vi "Change in Custom Actions.vi"(8 "error in (no error)":errorcluster, 10 "Custom Actions":T1[](array[typedef]), 11 "Bundle Builder in":refnum<class "Bundle Builder.lvclass">) -> (0 "error out":errorcluster, 1 "Custom Actions File Names":string[](array[string]), 2 "Product List File Names":string[](array[string]), 3 "Bundle Builder out":refnum<class "Bundle Builder.lvclass">, 4 "Bundle Filename":string)   [LabVIEW 2020, in "Bundle Builder.lvclass"]
uses:
  Bundle Builder.lvclass
  Typedef/Custom Action.ctl
  Bundle Builder.lvclass/Bundle Builder.ctl
  4f63f28f-5265-4602-8317-7e5f909f2807.vi
  5d65ce95-3f27-4ad9-b4d3-753b2ea8e44f.vi
  <vilib>/Comparison/Equal/Equal Functor/Equal Functor.lvclass
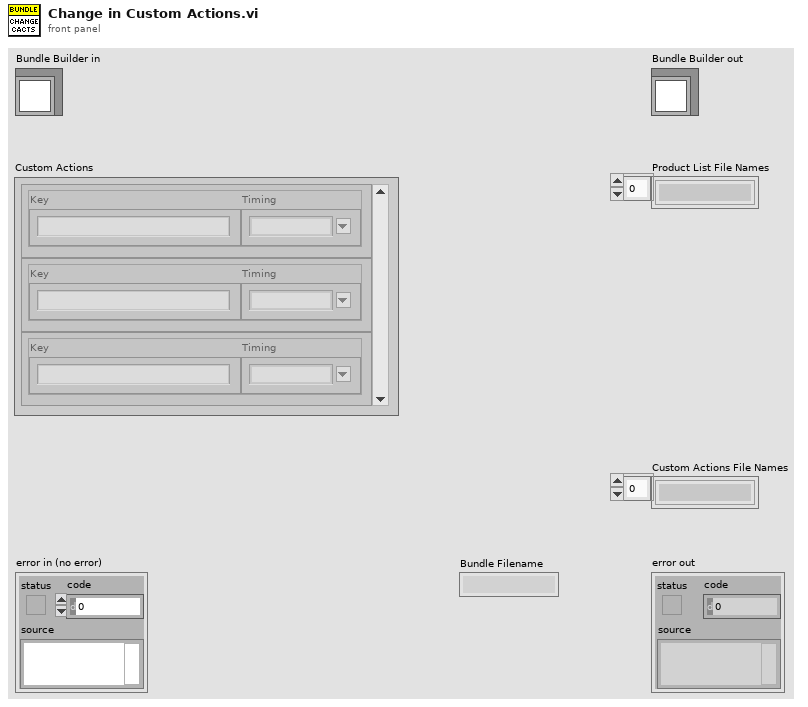
[diagram p1: front panel]
types:
  T1 = typedef "Custom Action.ctl" = cluster{"Key":string, "Timing":string}
  T2 = enum16{"All Elements Deleted", "Element Deleted", "Element Inserted", "Element Content Changed"}
  T3 = cluster{"Display Name":string, "Commands":cluster{"Path":string, "Parameters":string, "Successful Exit Codes":string}[]}[]
  T4 = cluster{"Display Name":string, "Commands":cluster{"Path":string, "Parameters":string, "Successful Exit Codes":string}[]}
  T5 = typedef "Custom Action Definition.ctl" = cluster{"Display Name":string, "Commands":cluster{"Path":string, "Parameters":string, "Successful Exit Codes":string}[]}
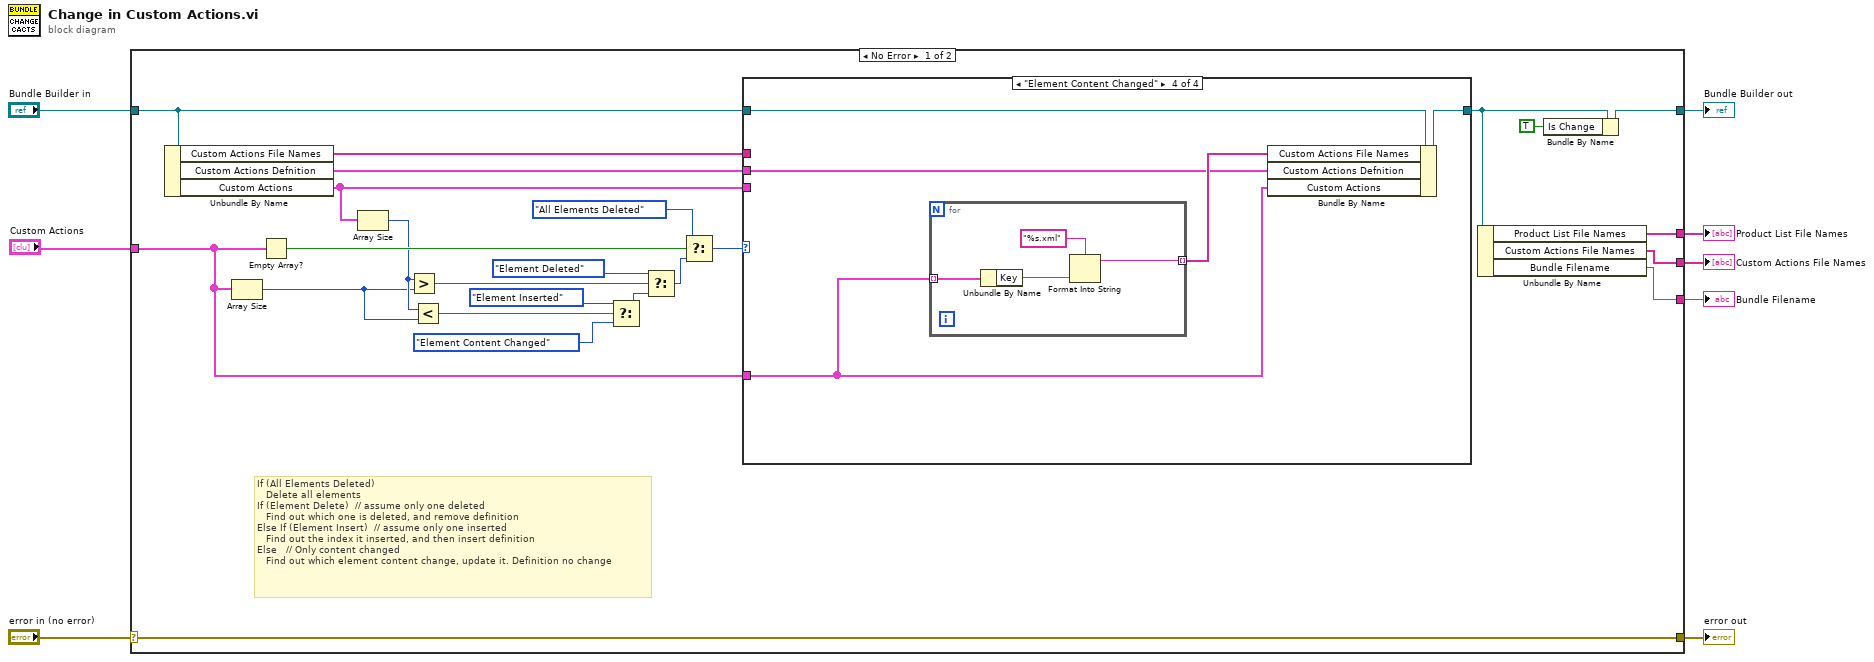
[diagram p0: block diagram]
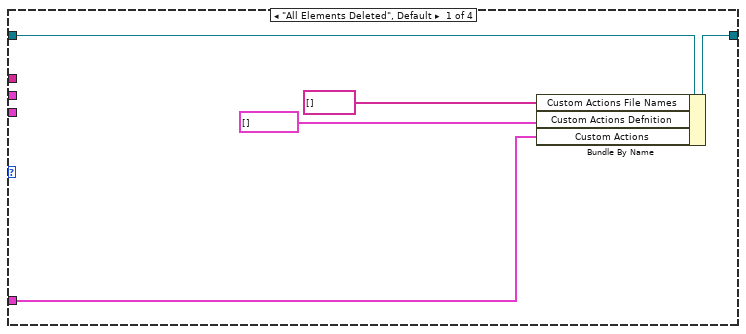
[diagram p2: hidden frame]
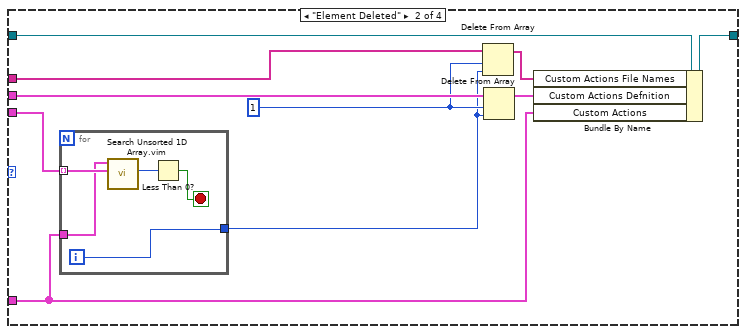
[diagram p3: hidden frame]
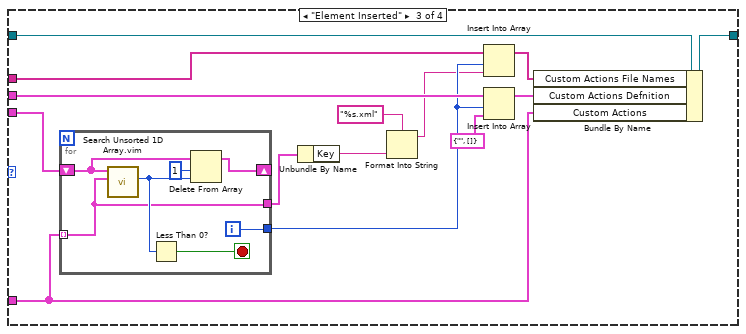
[diagram p4: hidden frame]
diagram:
  n1 = case shown="No Error" "error in (no error)" {
    selector: "error in (no error)" -> [w32 w84]
    tunnel: [w32 w84] -> w7
    tunnel: [w10 w83] -> w5
    tunnel: "Bundle Builder in" -> [w19 w83]
    tunnel: "Custom Actions" -> [w18 _]
    tunnel: [w13 _] -> w4
    tunnel: [w12 _] -> w3
    tunnel: [w11 _] -> w2
    frame No Error {
      # "If (All Elements Deleted)\n   Delete all elements\nIf (Element Delete)  // assume only one deleted\n   Find out which one is deleted, and remove definition\nElse If (Element Insert)  // assume only one inserted\n   Find out the index it inserted, and then insert definition\nElse   // Only content changed\n   Find out which element content change, update it. Definition no change"
      n2 = Unbundle By Name(w19) -> ("Custom Actions File Names"=w14:string[], "Custom Actions Defnition"=w16:T5[], "Custom Actions"=w17:T1[])
      n3 = Array Size(array=w18) -> (size(s)=w25:i32)
      n4 = Empty Array?(array=w18) -> (empty?=w31:bool)
      n5 = Array Size(array=w17) -> (size(s)=w26:i32)
      n6 = Greater?(x=w26, y=w25) -> (0:w27:bool)
      n7 = Less?(x=w26, y=w25) -> (x < y?=w22:bool)
      n8 = Select(t=T2."Element Inserted", s=w22, f=T2."Element Content Changed") -> (s? t:f=w24:T2)
      n9 = Select(t=T2."Element Deleted", s=w27, f=w24) -> (s? t:f=w28:T2)
      n10 = Select(t=T2."All Elements Deleted", s=w31, f=w28) -> (s? t:f=w20:T2)
      n11 = case shown="\"Element Content Changed\"" w20 {
        tunnel: w19 -> [w37 w47 w66 w78]
        tunnel: [w36 w46 w65 w77] -> w15
        tunnel: w18 -> [w35 w43 w62 w76]
        tunnel: w17 -> [_ w45 w64 _]
        tunnel: w16 -> [_ w44 w63 w74]
        tunnel: w14 -> [_ w42 w61 _]
        frame "All Elements Deleted", Default {
          n12 = Bundle By Name(cluster=w37, "Custom Actions File Names"=string[] [] ("Product List File Names"), "Custom Actions Defnition"=T3 [], "Custom Actions"=w35) -> (w36:refnum<class "Bundle Builder.lvclass">)
        }
        frame "Element Deleted" {
          w40 = 1 ("length")
          n13 = for {
            tunnel: w45 -> [w52] mode=indexing
            tunnel: w43 -> [w51]
            tunnel: [w48] -> w39
            i -> [w48]
            stop <- w50 stop-if-true
            n14 = call "Search Unsorted 1D Array.vim"("element"=w52, "unsorted 1D array"=w51) -> ("index of element"=w49:i32)  [unwired: 9 in]
            n15 = Less Than 0?(x=w49) -> (x < 0?=w50:bool)
          }
          n16 = Delete From Array(array=w42, length=w40, index=w39) -> (array with subset deleted=w41:string[])  [unwired: 1 out]
          n17 = Delete From Array(array=w44, length=w40, index=w39) -> (array with subset deleted=w38:T5[])  [unwired: 1 out]
          n18 = Bundle By Name(cluster=w47, "Custom Actions File Names"=w41, "Custom Actions Defnition"=w38, "Custom Actions"=w43) -> (w46:refnum<class "Bundle Builder.lvclass">)
        }
        frame "Element Inserted" {
          n19 = for {
            tunnel: w62 -> [w67] mode=indexing
            tunnel: [w72] -> w60
            shift-right: [w68] -> _
            shift-left: w64 -> [w71]
            tunnel: [w67] -> w59
            i -> [w72]
            stop <- w73 stop-if-true
            n20 = call "Search Unsorted 1D Array.vim"("element"=w67, "unsorted 1D array"=w71) -> ("index of element"=w70:i32)  [unwired: 9 in]
            n21 = Less Than 0?(x=w70) -> (x < 0?=w73:bool)
            n22 = Delete From Array(array=w71, length=1, index=w70) -> (array with subset deleted=w68:T1[])  [unwired: 1 out]
          }
          n23 = Unbundle By Name(w59) -> ("Key"=w57:string)
          n24 = Format Into String(format string="%s.xml", w57) -> (resulting string=w56:string)  [unwired: 2 in, 1 out]
          n25 = Insert Into Array(array=w61, index=w60, new element=w56) -> (w55:string[])
          n26 = Insert Into Array(array=w63, index=w60, new element=T4 {"Display Name"="", "Commands"=[]} ("Custom Actions")) -> (w54:T5[])
          n27 = Bundle By Name(cluster=w66, "Custom Actions File Names"=w55, "Custom Actions Defnition"=w54, "Custom Actions"=w62) -> (w65:refnum<class "Bundle Builder.lvclass">)
        }
        frame "Element Content Changed" {
          n28 = for {
            tunnel: w76 -> [w80] mode=indexing
            tunnel: [w79] -> w75 mode=indexing
            n29 = Unbundle By Name(w80) -> ("Key"=w81:string)
            n30 = Format Into String(format string="%s.xml", w81) -> (resulting string=w79:string)  [unwired: 2 in, 1 out]
          }
          n31 = Bundle By Name(cluster=w78, "Custom Actions File Names"=w75, "Custom Actions Defnition"=w74, "Custom Actions"=w76) -> (w77:refnum<class "Bundle Builder.lvclass">)
        }
      }
      n32 = Unbundle By Name(w15) -> ("Product List File Names"=w13:string[], "Custom Actions File Names"=w12:string[], "Bundle Filename"=w11:string)
      n33 = Bundle By Name(cluster=w15, "Is Change"=TRUE) -> (w10:refnum<class "Bundle Builder.lvclass">)
    }
    frame Error {
    }
  }
  "error out" <- w7
  "Bundle Builder out" <- w5
  "Product List File Names" <- w4
  "Custom Actions File Names" <- w3
  "Bundle Filename" <- w2
